vi "Fill From.vi"(5 "Col":i32, 6 "Attributes":T1, 8 "error in (no error)":errorcluster, 10 "Char":string, 11 "TermLine in":refnum<class "TermLine.lvclass">) -> (0 "error out":errorcluster, 3 "TermLine out":refnum<class "TermLine.lvclass">)   [LabVIEW 2020, in "Terminal.lvlib" / "TermLine.lvclass"]
uses:
  TermLine.lvclass
  TermLine.lvclass/TermLine.ctl
  Term Char.ctl
  Terminal.lvlib
  Text Attributes.ctl
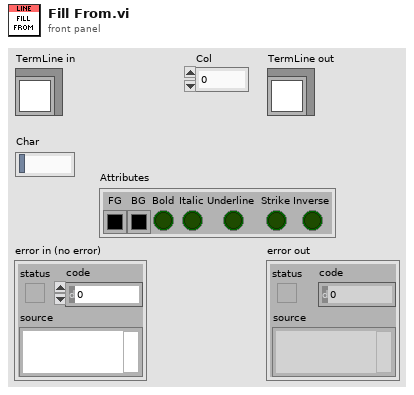
[diagram p1: front panel]
types:
  T1 = typedef "Terminal.lvlib/Text Attributes.ctl" = cluster{"FG":u32, "BG":u32, "Bold":bool, "Italic":bool, "Underline":bool, "Strike":bool, "Inverse":bool}
  T2 = typedef "Terminal.lvlib/Term Char.ctl" = cluster{"Char":string, "Attributes":T1}
  T3 = typedef "Terminal.lvlib/TermLine.lvclass/Ref Data.ctl" = cluster{"Chars":T2[], "Width":i32}
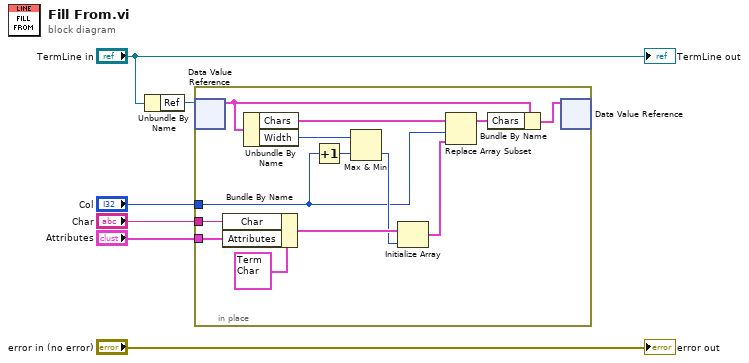
[diagram p0: block diagram]
diagram:
  n1 = Unbundle By Name("TermLine in") -> ("Ref"=w5:refnum<data-value>)
  n2 = in-place {
    in-place-border: "Col" -> [w9]
    in-place-border: "Char" -> [w16]
    in-place-border: "Attributes" -> [w7]
    n3 = in-place-dvr #1(w5) -> (w19:T3)  [unwired: 1 out]
    n4 = Bundle By Name(cluster=T2 {"Char"=" ", "Attributes"={"FG"=16777216, "BG"=16777216, "Bold"=FALSE, "Italic"=FALSE, "Underline"=FALSE, "Strike"=FALSE, "Inverse"=FALSE}} ("Term Char"), "Char"=w16, "Attributes"=w7) -> (w14:T2)
    n5 = Unbundle By Name(w19) -> ("Chars"=w11:T2[], "Width"=w15:i32)
    n6 = Increment(x=w9) -> (x+1=w13:i32)
    n7 = Max & Min(x=w15, y=w13) -> (min(x,y)=w12:i32)  [unwired: 1 out]
    n8 = Initialize Array(w14, w12) -> (w10:T2[])
    n9 = Replace Array Subset(array=w11, new element=w10, index=w9) -> (w8:T2[])
    n10 = Bundle By Name(cluster=w19, "Chars"=w8) -> (w18:T3)
    n11 = in-place-dvr #1(w18) -> ()  [unwired: 2 out]
  }
  "error out" <- "error in (no error)"
  "TermLine out" <- "TermLine in"
